vi "Create.vi"(10 "Events":T1) -> (3 "Status Updater out":refnum<class "Status Events.lvclass">)   [LabVIEW 2014, in "Status Events.lvclass"]
uses:
  Status Events.lvclass
  Status Events.lvclass/Status Events.ctl
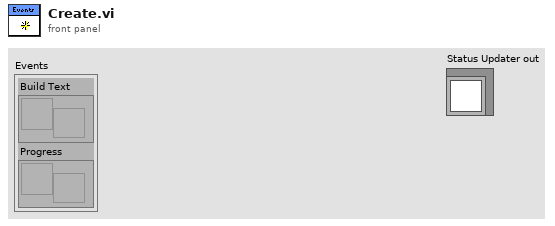
[diagram p1: front panel]
types:
  T1 = cluster{"Build Text":refnum<user-event>, "Progress":refnum<user-event>}
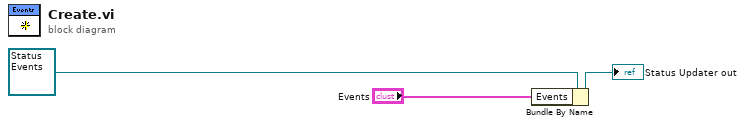
[diagram p0: block diagram]
diagram:
  n1 = Bundle By Name(cluster=refnum<class "Status Events.lvclass"> refnum ("Status Updater in"), "Events"="Events") -> (→"Status Updater out":refnum<class "Status Events.lvclass">)
